vi "GetControlReferenceFromTabControl.vi"(8 "error in (no error)":errorcluster, 9 "control":i32, 10 "page":i32, 11 "Ctl Refnum":refnum<vi>) -> (0 "error out":errorcluster, 3 "element":refnum<vi>)   [LabVIEW 2016]
panel:
  in  "TabCtl Refnum":refnum<vi>
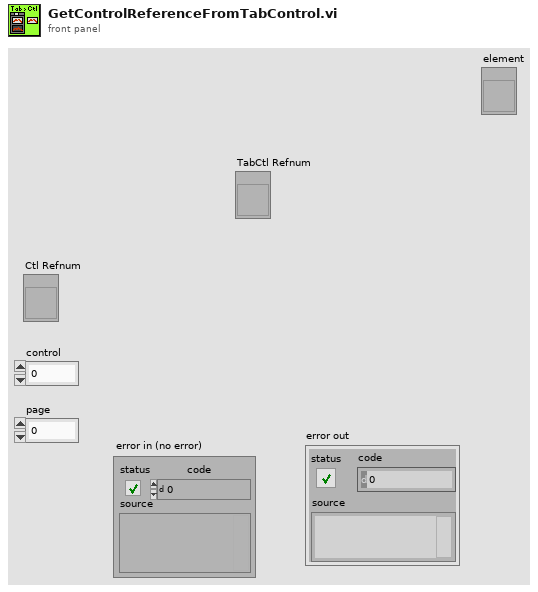
[diagram p1: front panel]
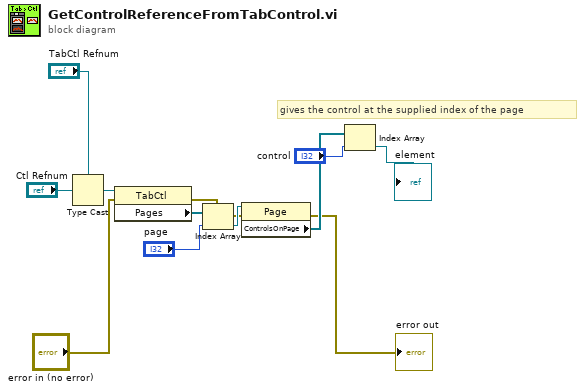
[diagram p0: block diagram]
diagram:
  # "gives the control at the supplied index of the page"
  n1 = Type Cast(type="TabCtl Refnum", x="Ctl Refnum") -> (*(type *) &x=w6:refnum<vi>)
  n2 = property class="TabCtl"(reference=w6, error in="error in (no error)") -> (error out=w2:errorcluster, "Pages"=w7:refnum<vi>[])  [unwired: 1 out]
  n3 = Index Array(array=w7, index="page") -> (element=w9:refnum<vi>)
  n4 = property class="Page"(reference=w9, error in=w2) -> (error out=→"error out":errorcluster, "ControlsOnPage"=w11:refnum<vi>[])  [unwired: 1 out]
  n5 = Index Array(array=w11, index="control") -> (element=→"element":refnum<vi>)
